vi "Set Serial Settings.vi"(5 "serial type":T2, 6 "parity (even)":T1=2 items=["None", "Odd", "Even", "Mark", "Space"], 7 "flow control (none)":T3 items=["None", "XON/XOFF", "RTS/CTS", "XON/XOFF & RTS/CTS", "DTR/DSR", "XON/XOFF & DTR/DSR"], 8 "error in (no error)":errorcluster, 9 "baud rate":u32=9600, 10 "VISA resource name":refnum<visa-resource-name>, 11 "Item Ref in":T4 format="%.0x") -> (0 "error out":errorcluster, 3 "Item Ref out":T4 format="%.0x")   [LabVIEW 2015, in "Modbus Master System Explorer.lvlib"]
uses:
  Modbus Master System Explorer.lvlib
  <vilib>/NI Veristand/Custom Device API/Custom Device Item Ref.ctl
  Shared/Controls/Flow Control.ctl
  Shared/Controls/Serial Type.ctl
  Shared/Controls/Parity.ctl
  Shared/Constants.vi
  <vilib>/NI Veristand/Custom Device API/Set Item Property (String).vi
  <vilib>/NI Veristand/Custom Device API/Set Item Property (U32).vi
  <vilib>/NI Veristand/Custom Device API/Set Item Property (U16).vi
  <vilib>/NI VeriStand/Custom Device API/Custom Device API.lvlib
  Shared/Modbus Master Shared.lvlib
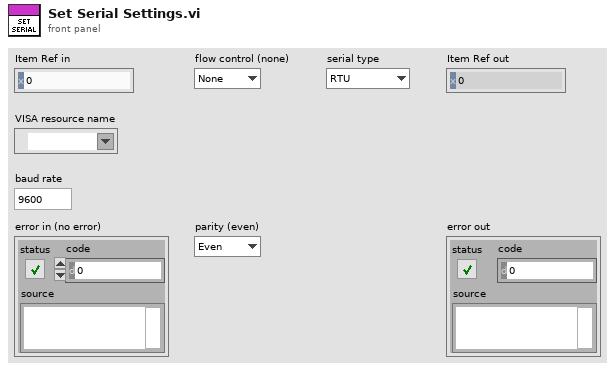
[diagram p1: front panel]
types:
  T1 = typedef "Modbus Master Shared.lvlib/Parity.ctl" = u16
  T2 = typedef "Modbus Master Shared.lvlib/Serial Type.ctl" = enum16{"RTU", "ASCII"}
  T3 = typedef "Modbus Master Shared.lvlib/Flow Control.ctl" = u16
  T4 = typedef "Custom Device API.lvlib/Custom Device Item Ref.ctl" = u64
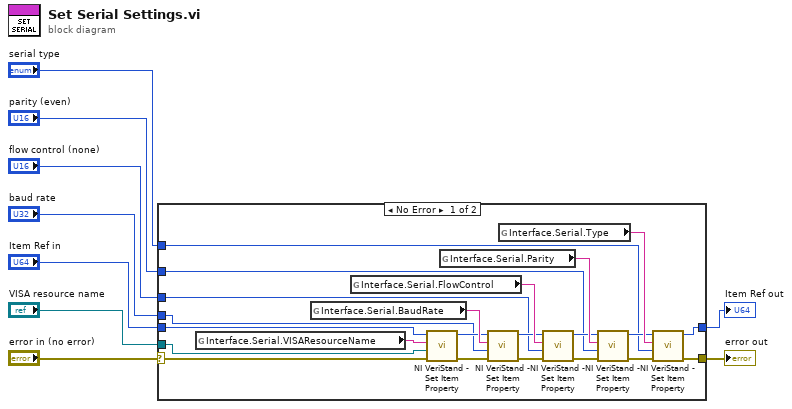
[diagram p0: block diagram]
diagram:
  n1 = case shown="No Error" "error in (no error)" {
    selector: "error in (no error)" -> [w17 w32]
    tunnel: [w31 w32] -> w9
    tunnel: [w30 w33] -> w8
    tunnel: "Item Ref in" -> [w16 w33]
    tunnel: "VISA resource name" -> [w15 _]
    tunnel: "baud rate" -> [w14 _]
    tunnel: "flow control (none)" -> [w13 _]
    tunnel: "parity (even)" -> [w12 _]
    tunnel: "serial type" -> [w11 _]
    frame No Error {
      n2 = global read "Constants.vi" "Interface.Serial.VISAResourceName"() -> (w10:string)
      n3 = global read "Constants.vi" "Interface.Serial.BaudRate"() -> (w20:string)
      n4 = global read "Constants.vi" "Interface.Serial.FlowControl"() -> (w23:string)
      n5 = call-poly <vilib>:"NI VeriStand - Set Item Property.vi"("error in (no error)"=w17, "Value"=w15, "Property Name"=w10, "Item Ref in"=w16) -> ("error out"=w18:errorcluster, "Item Ref out"=w19:T4)  [unwired: 5 in, 1 out]
      n6 = global read "Constants.vi" "Interface.Serial.Parity"() -> (w26:string)
      n7 = call-poly <vilib>:"NI VeriStand - Set Item Property.vi"("error in (no error)"=w18, "Value"=w14, "Property Name"=w20, "Item Ref in"=w19) -> ("error out"=w21:errorcluster, "Item Ref out"=w22:T4)  [unwired: 5 in, 1 out]
      n8 = global read "Constants.vi" "Interface.Serial.Type"() -> (w29:string)
      n9 = call-poly <vilib>:"NI VeriStand - Set Item Property.vi"("error in (no error)"=w21, "Value"=w13, "Property Name"=w23, "Item Ref in"=w22) -> ("error out"=w24:errorcluster, "Item Ref out"=w25:T4)  [unwired: 5 in, 1 out]
      n10 = call-poly <vilib>:"NI VeriStand - Set Item Property.vi"("error in (no error)"=w24, "Value"=w12, "Property Name"=w26, "Item Ref in"=w25) -> ("error out"=w27:errorcluster, "Item Ref out"=w28:T4)  [unwired: 5 in, 1 out]
      n11 = call-poly <vilib>:"NI VeriStand - Set Item Property.vi"("error in (no error)"=w27, "Value"=w11, "Property Name"=w29, "Item Ref in"=w28) -> ("error out"=w31:errorcluster, "Item Ref out"=w30:T4)  [unwired: 5 in, 1 out]
    }
    frame Error {
    }
  }
  "error out" <- w9
  "Item Ref out" <- w8
